vi "GetFileHexapod.vi"(4 "error in":errorcluster, 6 "HexpodFileName":string, 7 "Projet":string) -> (0 "error out":errorcluster, 2 "LocalHexapodFile":path, 3 "ProjetOut":string)   [LabVIEW 2017]
uses:
  DefDeType/WhichPath.ctl
panel:
  out "file or folder exists?":bool
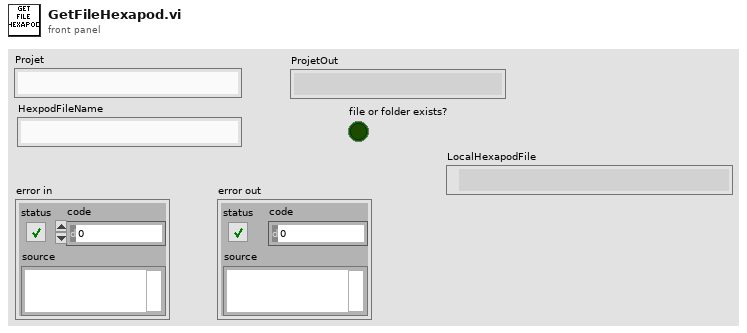
[diagram p1: front panel]
types:
  T1 = typedef "WhichPath.ctl" = enum16{"DossierProjet", "Config", "Meas", "MeasSuitCase", "MeasOnBoard", "MeasQualisys", "MeasTDMS", "MeasHexapode", "MeasNortek", "Fig", "Res", "MeasUSB"}
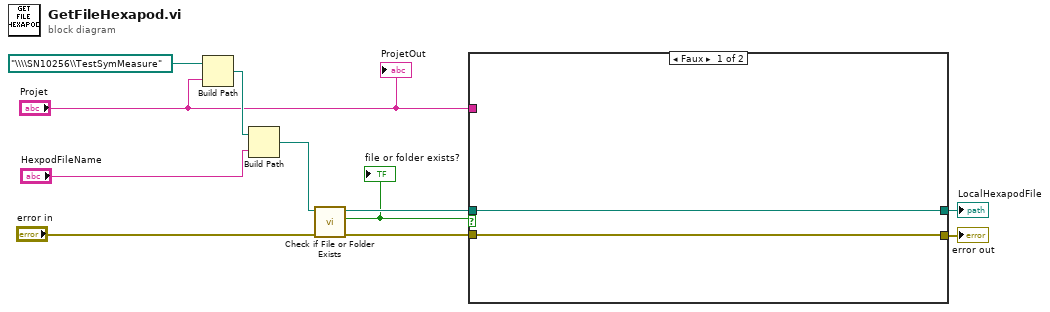
[diagram p0: block diagram]
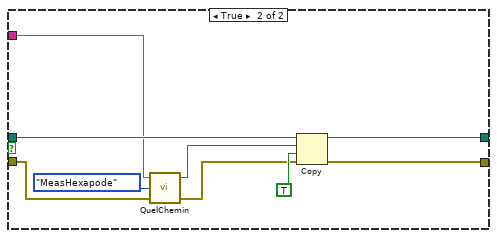
[diagram p2: hidden frame]
diagram:
  n1 = Build Path(base path=path "\\\\SN10256\\TestSymMeasure" ("CheminDepartFichierHExapode"), name or relative path="Projet") -> (appended path=w9:path)
  n2 = Build Path(base path=w9, name or relative path="HexpodFileName") -> (appended path=w7:path)
  n3 = call <vilib>:"Check if File or Folder Exists.vi"("error in (no error)"="error in", "path"=w7) -> ("error out"=w6:errorcluster, "file or folder exists?"=w4:bool, "dup path"=w5:path)  [unwired: 7 in]
  "file or folder exists?" <- w4
  n4 = case shown="Faux" w4 {
    tunnel: w6 -> [w13 w20]
    tunnel: w5 -> [w12 w22]
    tunnel: "Projet" -> [_ w18]
    tunnel: [w13 w15] -> w2
    tunnel: [w12 w14] -> w1
    frame False {
    }
    frame True {
      n5 = call "QuelChemin.vi"("Entrée d'erreur"=w20, "WhichPath?"=WhichPath."MeasHexapode", "NomProjet"=w18) -> ("Sortie d'erreur"=w19:errorcluster, "SurDisqueLocal"=w16:path)  [unwired: 1 out]
      n6 = Copy(8:w19, 9:TRUE ("overwrite (F)"), 10:w16, 11:w22) -> (0:w15:errorcluster, 3:w14:path)  [unwired: 1 in, 1 out]
    }
  }
  "error out" <- w2
  "LocalHexapodFile" <- w1
  "ProjetOut" <- "Projet"
